vi "Simple Control.vi"() -> ()   [LabVIEW 2014]
uses:
  <vilib>/LVH/AR Drone Toolkit/AR Drone.lvlib
panel:
  in  "stop":bool
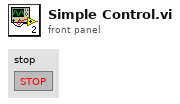
[diagram p1: front panel]
types:
  T1 = typedef "AR Drone.lvlib/AR Drone Resource.ctl" = cluster{"UDP Control Connection":refnum<k16>, "UDP NavData Connection":refnum<k16>, "UDP Video Connection (Drone 1.0)":refnum<k16>, "TCP Video Connection (Drone 2.0)":refnum<k5>, "TCP Control Port Connection":refnum<k5>, "Drone IP address":string, "Drone Command Port":u16, "Drone NavData Port":u16, "Drone Vid Stream Port":u16, "Drone TCP Control Port":u16, "Home IP address":string, "Home Command Port":u16, "Home NavData Port":u16, "Home Vid Stream Port":u16, "Drone Version":i32}
  T2 = cluster{"Roll":sgl, "Pitch":sgl, "Vertical Speed":sgl, "Yaw Speed":sgl}
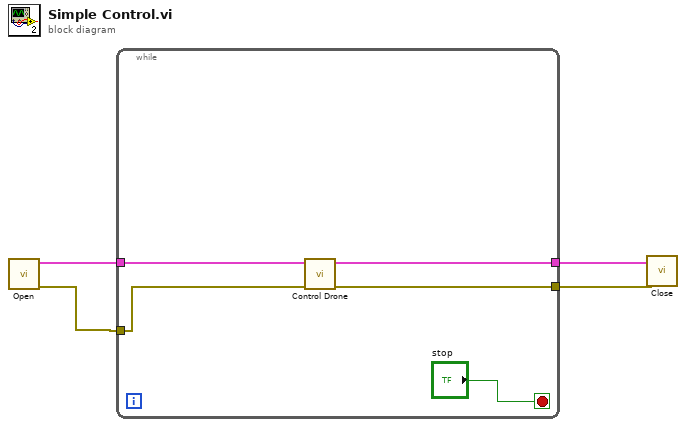
[diagram p0: block diagram]
diagram:
  n1 = call <vilib>:"Open.vi"() -> ("error out"=w3:errorcluster, "AR Drone Resource"=w4:T1)  [unwired: 10 in]
  n2 = while {
    tunnel: w4 -> [w8]
    tunnel: w3 -> [w7]
    tunnel: [w10] -> w2
    tunnel: [w9] -> w1
    stop <- "stop" stop-if-true
    n3 = call <vilib>:"Control Drone.vi"("error in (no error)"=w7, "AR Drone Resource"=w8) -> ("error out"=w9:errorcluster, "AR Drone Resource Out"=w10:T1, "Control Cluster"=w6:T2)  [unwired: 7 in]
  }
  n4 = call <vilib>:"Close.vi"("error in (no error)"=w1, "AR Drone Resource"=w2) -> ()  [unwired: 9 in, 1 out]
